vi "AVI-file management logic.vi"(8 "error in (no error)":errorcluster, 11 "First AVI2 video's Path":path) -> (0 "error out":errorcluster, 1 "A non .avi file was selected, or no extension present":bool, 2 "Empty or not a path or not a \".avi\" file or error":bool, 3 "filename without extension":string)   [LabVIEW 2020]
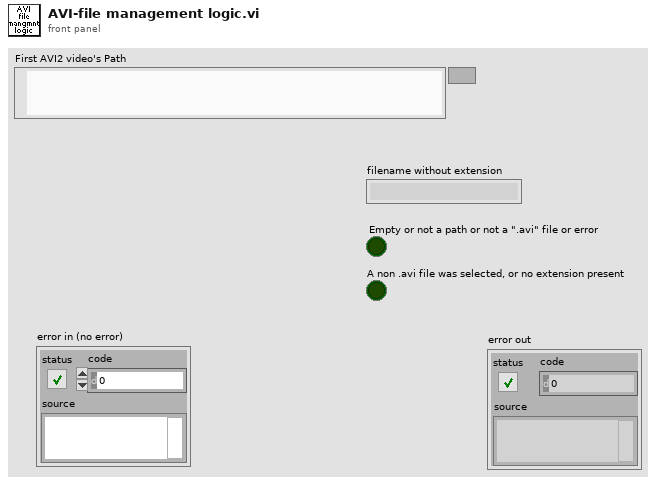
[diagram p1: front panel]
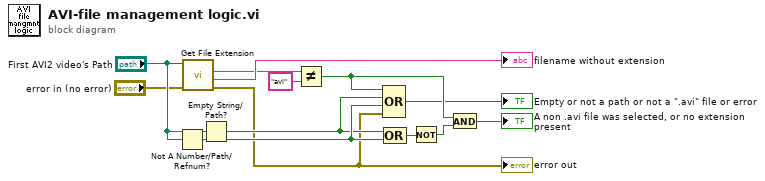
[diagram p0: block diagram]
diagram:
  n1 = Not A Number/Path/Refnum?(number/path/refnum="First AVI2 video's Path") -> (NaN/Path/Refnum?=w11:bool)
  n2 = call <vilib>:"Get File Extension.vi"("error in (no error)"="error in (no error)", "file"="First AVI2 video's Path") -> ("error out"=w1:errorcluster, "filename without extension"=→"filename without extension":string, "lowercase file extension"=w5:string)  [unwired: 5 in, 2 out]
  "error out" <- w1
  n3 = Empty String/Path?(string/path="First AVI2 video's Path") -> (empty?=w10:bool)
  n4 = Not Equal?(x=w5, y="avi") -> (x != y?=w12:bool)
  n5 = Compound Arithmetic op=OR(w12, w10, w11, w1) -> (→"Empty or not a path or not a \".avi\" file or error":bool)
  n6 = Compound Arithmetic op=OR(w10, w11) -> (w9:bool)
  n7 = Not(x=w9) -> (.not. x?=w8:bool)
  n8 = And(x=w12, y=w8) -> (x .and. y?=→"A non .avi file was selected, or no extension present":bool)
